vi "CThread For Loop.vi"   [LabVIEW 2012, in "CThread.lvlib"]
uses:
  CThread.lvlib
  XNodes/terminalnode/CThread VI Terminal Node.xnode
  Core/CThread Thread Properties.ctl
  CRef/Interface/CRef Boolean.llb/Boolean CReference.ctl
  CRef/CRef.lvlib
  CRef/Interface/CRef Numeric.llb/I32 CReference.ctl
  Base/CThread Base - For Loop.vi
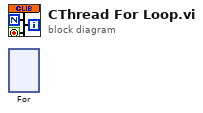
[diagram p0: block diagram]
diagram:
  n1 = xnode "For"() -> ()  [unwired: 4 in, 2 out]
